vi "niDTS GNSS Dut Rx Abort.vi"(0 "Dut Handle in":T1, 11 "error in (no error)":errorcluster) -> (4 "Dut Handle out":T1, 15 "error out":errorcluster)   [LabVIEW 2015, in "niDTS GNSS.lvlib"]
uses:
  niDTS GNSS.lvlib
  Framework/Dut/Includes/niDTS Dut INC Handle.ctl
  Framework/Dut/Objects/BASE_class/niDTS Dut.lvclass
  Includes/niDTS GNSS Dut INC Handle.ctl
  Objects/BASE_class/niDTS GNSS Dut.lvclass
  Framework/niDTS Framework.lvlib
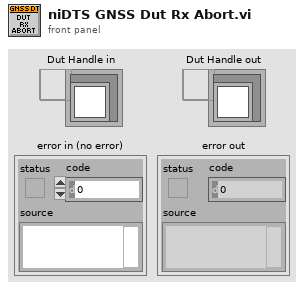
[diagram p1: front panel]
types:
  T1 = typedef "niDTS Framework.lvlib/niDTS Dut INC Handle.ctl" = refnum<data-value>
  T2 = typedef "niDTS GNSS.lvlib/niDTS GNSS Dut INC Handle.ctl" = refnum<data-value>
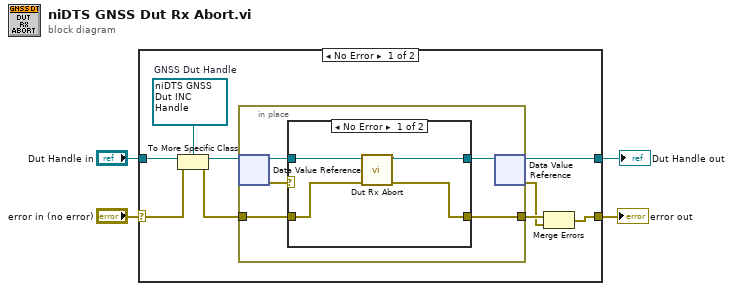
[diagram p0: block diagram]
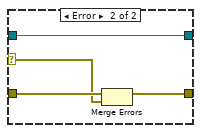
[diagram p2: hidden frame]
diagram:
  n1 = case shown="No Error" "error in (no error)" {
    selector: "error in (no error)" -> [w5 w27]
    tunnel: "Dut Handle in" -> [w13 w28]
    tunnel: [w12 w28] -> w3
    tunnel: [w7 w27] -> w2
    frame No Error {
      w9 = T2 refnum  # GNSS Dut Handle
      n2 = To More Specific Class(target class=w9, reference=w13, error in=w5) -> (specific class reference=w11:T2, error out=w10:errorcluster)
      n3 = in-place {
        in-place-border: w10 -> [w15]
        in-place-border: [w14] -> w8
        n4 = in-place-dvr #1(w11) -> (w17:refnum<class "niDTS GNSS Dut.lvclass">, w18:errorcluster)
        n5 = case shown="No Error" w18 {
          selector: w18 -> [_ w24]
          tunnel: w17 -> [w22 w26]
          tunnel: [w21 w26] -> w16
          tunnel: w15 -> [w20 w25]
          tunnel: [w19 w23] -> w14
          frame No Error {
            n6 = call-dynamic "Dut Rx Abort.vi"("niDTS DUT in"=w22, "error in (no error)"=w20) -> ("niDTS DUT out"=w21:refnum<class "niDTS GNSS Dut.lvclass">, "error out"=w19:errorcluster)  [unwired: 12 in]
          }
          frame Error {
            n7 = Merge Errors(w25, w24) -> (w23:errorcluster)
          }
        }
        n8 = in-place-dvr #1(w16) -> (w12:T2, w6:errorcluster)
      }
      n9 = Merge Errors(w8, w6) -> (w7:errorcluster)
    }
    frame Error {
    }
  }
  "Dut Handle out" <- w3
  "error out" <- w2
